vi "Exit Loop.vi"(0 "Diagram in":refnum<vi>, 1 "Loop Terminal Types":T1[](array[typedef]), 5 "Outputs":refnum<vi>[](array[refnum]), 7 "Shift Registers":refnum<vi>[](array[refnum]), 9 "Conditional Terminals":refnum<vi>[](array[refnum]), 11 "error in (no error)":errorcluster) -> (4 "Diagram out":refnum<vi>, 6 "Outputs":refnum<vi>[](array[refnum]), 8 "Shift Registers":refnum<vi>[](array[refnum]), 15 "error out":errorcluster)   [LabVIEW 2015, in "Scripting.lvlib"]
uses:
  Scripting.lvlib
  Loop Terminal Type.ctl
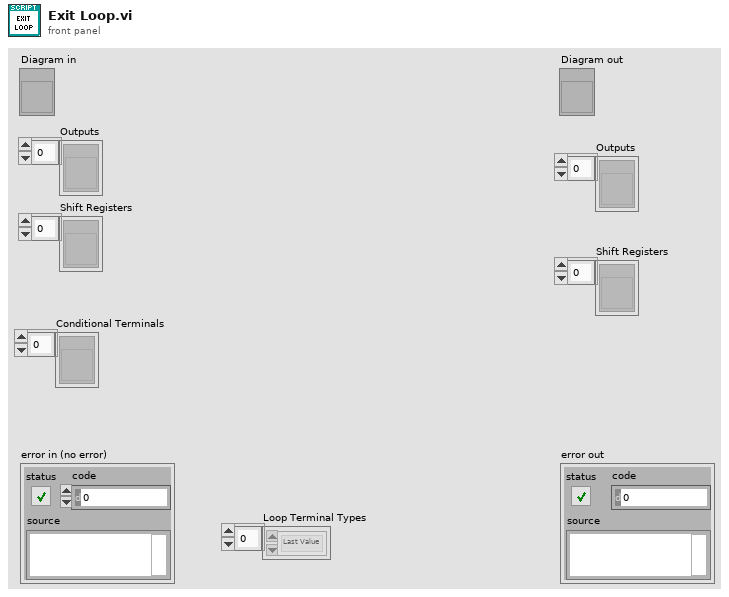
[diagram p1: front panel]
types:
  T1 = typedef "Scripting.lvlib/Loop Terminal Type.ctl" = enum16{"Last Value", "Indexing", "Concatenating"}
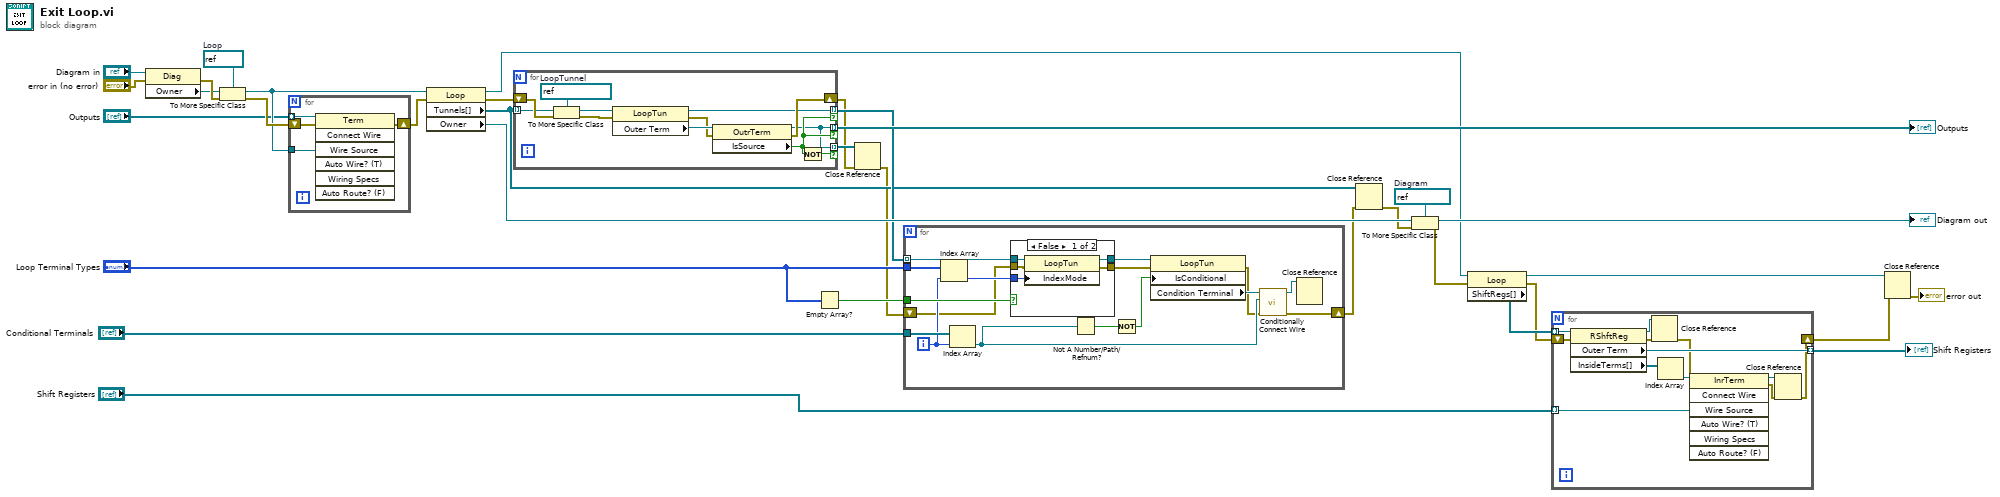
[diagram p0: block diagram]
diagram:
  w29 = refnum<vi> refnum  # Diagram
  w31 = refnum<vi> refnum  # Loop
  n1 = property class="Diag"(reference="Diagram in", error in="error in (no error)") -> (error out=w32:errorcluster, "Owner"=w30:refnum<vi>)  [unwired: 1 out]
  n2 = To More Specific Class(target class=w31, reference=w30, error in=w32) -> (specific class reference=w28:refnum<vi>, error out=w33:errorcluster)
  n3 = for {
    tunnel: w28 -> [w36]
    shift-right: [w35] -> w27
    shift-left: w33 -> [w37]
    tunnel: "Outputs" -> [w34] mode=indexing
    n4 = invoke class="Term" method="Connect Wire"(reference=w34, error in=w37, "Wire Source"=w36) -> (error out=w35:errorcluster)  [unwired: 4 in, 6 out]
  }
  n5 = property class="Loop"(reference=w28, error in=w27) -> (reference out=w8:refnum<vi>, error out=w19:errorcluster, "Tunnels[]"=w6:refnum<vi>[], "Owner"=w20:refnum<vi>)
  n6 = for {
    tunnel: w6 -> [w44] mode=indexing
    tunnel: [w39] -> w22 mode=indexing if=w40
    shift-right: [w46] -> w2
    shift-left: w19 -> [w49]
    tunnel: [w41] -> w13 mode=indexing if=w40
    tunnel: [w39] -> w3 mode=indexing if=w38
    w42 = refnum<vi> refnum  # LoopTunnel
    n7 = To More Specific Class(target class=w42, reference=w44, error in=w49) -> (specific class reference=w43:refnum<vi>, error out=w45:errorcluster)
    n8 = property class="LoopTun"(reference=w43, error in=w45) -> (reference out=w41:refnum<vi>, error out=w47:errorcluster, "Outer Term"=w48:refnum<vi>)
    n9 = property class="OutrTerm"(reference=w48, error in=w47) -> (reference out=w39:refnum<vi>, error out=w46:errorcluster, "IsSource"=w40:bool)
    n10 = Not(x=w40) -> (.not. x?=w38:bool)
  }
  "Outputs" <- w22
  n11 = Empty Array?(array="Loop Terminal Types") -> (empty?=w11:bool)
  n12 = Close Reference(reference=w3, error in (no error)=w2) -> (error out=w1:errorcluster)
  n13 = for {
    tunnel: w13 -> [w65] mode=indexing
    tunnel: "Loop Terminal Types" -> [w63]
    tunnel: w11 -> [w61]
    tunnel: "Conditional Terminals" -> [w60]
    shift-right: [w50] -> w5
    shift-left: w1 -> [w58]
    i -> [w59]
    n14 = Index Array(array=w63, index=w59) -> (element=w62:T1)
    n15 = Index Array(array=w60, index=w59) -> (element=w53:refnum<vi>)
    n16 = case shown="False" w61 {
      tunnel: w65 -> [w70 w72]
      tunnel: [w69 w72] -> w64
      tunnel: w62 -> [w68 _]
      tunnel: w58 -> [w67 w71]
      tunnel: [w66 w71] -> w57
      frame False {
        n17 = property class="LoopTun"(reference=w70, error in=w67, "IndexMode"=w68) -> (reference out=w69:refnum<vi>, error out=w66:errorcluster)
      }
      frame True {
      }
    }
    n18 = Not A Number/Path/Refnum?(number/path/refnum=w53) -> (NaN/Path/Refnum?=w56:bool)
    n19 = Not(x=w56) -> (.not. x?=w55:bool)
    n20 = property class="LoopTun"(reference=w64, error in=w57, "IsConditional"=w55) -> (error out=w52:errorcluster, "Condition Terminal"=w54:refnum<vi>)  [unwired: 1 out]
    n21 = call "Conditionally Connect Wire.vi"("error in (no error)"=w52, "Wire Source"=w53, "Terminal in"=w54) -> ("error out"=w50:errorcluster, "Terminal out"=w51:refnum<vi>)  [unwired: 7 in]
    n22 = Close Reference(reference=w51) -> ()  [unwired: 1 in, 1 out]
  }
  n23 = Close Reference(reference=w6, error in (no error)=w5) -> (error out=w4:errorcluster)
  n24 = To More Specific Class(target class=w29, reference=w20, error in=w4) -> (specific class reference=→"Diagram out":refnum<vi>, error out=w15:errorcluster)
  n25 = property class="Loop"(reference=w8, error in=w15) -> (reference out=w7:refnum<vi>, error out=w17:errorcluster, "ShiftRegs[]"=w18:refnum<vi>[])
  n26 = for {
    tunnel: w18 -> [w84] mode=indexing
    shift-right: [w74] -> w14
    shift-left: w17 -> [w81]
    tunnel: "Shift Registers" -> [w78] mode=indexing
    tunnel: [w77] -> w9 mode=indexing
    n27 = property class="RShftReg"(reference=w84, error in=w81) -> (reference out=w75:refnum<vi>, error out=w80:errorcluster, "Outer Term"=w77:refnum<vi>, "InsideTerms[]"=w83:refnum<vi>[])
    n28 = Close Reference(reference=w75, error in (no error)=w80) -> (error out=w76:errorcluster)
    n29 = Index Array(array=w83) -> (element=w82:refnum<vi>)  [unwired: 1 in]
    n30 = invoke class="InrTerm" method="Connect Wire"(reference=w82, error in=w76, "Wire Source"=w78) -> (reference out=w73:refnum<vi>, error out=w79:errorcluster)  [unwired: 4 in, 5 out]
    n31 = Close Reference(reference=w73, error in (no error)=w79) -> (error out=w74:errorcluster)
  }
  "Shift Registers" <- w9
  n32 = Close Reference(reference=w7, error in (no error)=w14) -> (error out=→"error out":errorcluster)
